vi "make_axes_caption.vi"(7 "Caption Properties":T2={"Show Captions"={"Show X Caption"=FALSE, "Show Z Caption"=TRUE, "Show Y Caption"=TRUE, "Show Opposite X Caption"=FALSE, "Show Opposite Y Caption"=TRUE, "Show Opposite Z Caption"=TRUE}, "Captions"={"Caption X"="", "Caption Y"="", "Caption Z"=""}, "Caption Color"={"Color X"=0, "Color Y"=0, "Color Z"=0}, "Caption Font Size"={"Font Size X"=12, "Font Size Y"=12, "Font Size Z"=12}}, 8 "Length":dbl, 9 "View Direction":T1(ring), 10 "Label Width":T3, 11 "Scene Object In":refnum<vi>) -> (3 "Scene Object Out":refnum<vi>)   [LabVIEW 2020, in "3DPC_SurfacePlot.xctl"]
uses:
  <vilib>/Native 3D Graph/xcontrol/3DPC_SurfacePlot.xctl
  <vilib>/Native 3D Graph/typedefs/prop_axes_captions.ctl
  <vilib>/Utility/miscctls.llb/LV3DPointTypeDef.ctl
  <vilib>/picture/3D Picture Control/Object/Create Object (name).vi
  <vilib>/picture/3D Picture Control/NI_3D Picture Control.lvlib
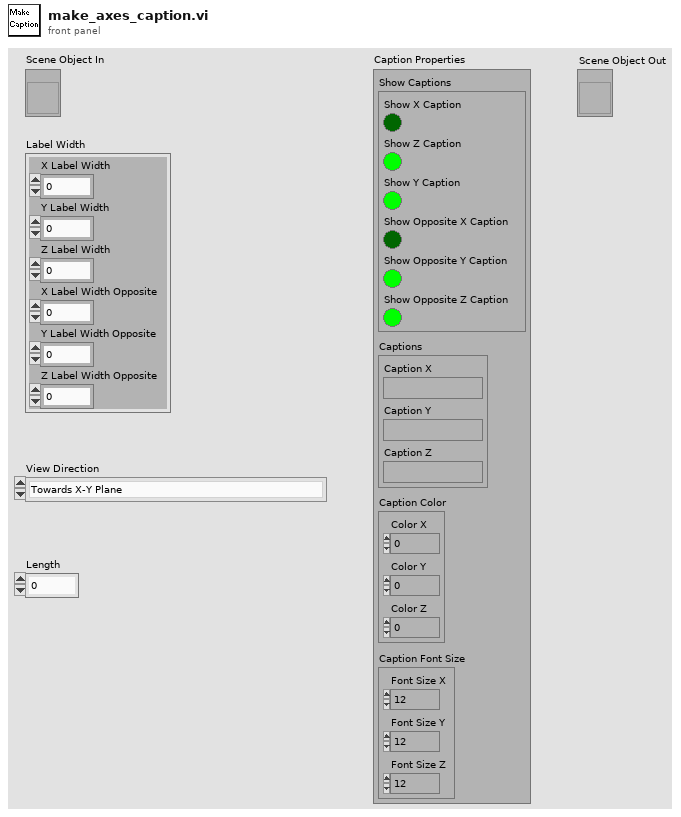
[diagram p1: front panel]
types:
  T1 = enum32{"Towards X-Y Plane", "Towards Y-Z Plane", "Towards X-Z Plane", "User Define"}
  T2 = typedef "3DPC_SurfacePlot.xctl/prop_axes_captions.ctl" = cluster{"Show Captions":cluster{"Show X Caption":bool, "Show Z Caption":bool, "Show Y Caption":bool, "Show Opposite X Caption":bool, "Show Opposite Y Caption":bool, "Show Opposite Z Caption":bool}, "Captions":cluster{"Caption X":string, "Caption Y":string, "Caption Z":string}, "Caption Color":cluster{"Color X":u32, "Color Y":u32, "Color Z":u32}, "Caption Font Size":cluster{"Font Size X":i16, "Font Size Y":i16, "Font Size Z":i16}}
  T3 = cluster{"X Label Width":dbl, "Y Label Width":dbl, "Z Label Width":dbl, "X Label Width Opposite":dbl, "Y Label Width Opposite":dbl, "Z Label Width Opposite":dbl}
  T4 = cluster{"Show X Caption":bool, "Show Z Caption":bool, "Show Y Caption":bool, "Show Opposite X Caption":bool, "Show Opposite Y Caption":bool, "Show Opposite Z Caption":bool}
  T5 = cluster{"Caption X":string, "Caption Y":string, "Caption Z":string}
  T6 = cluster{"Font Size X":i16, "Font Size Y":i16, "Font Size Z":i16}
  T7 = cluster{"Font Size X":dbl, "Font Size Y":dbl, "Font Size Z":dbl}
  T8 = typedef "LV3DPointTypeDef.ctl" = cluster{"X":sgl, "Y":sgl, "Z":sgl}
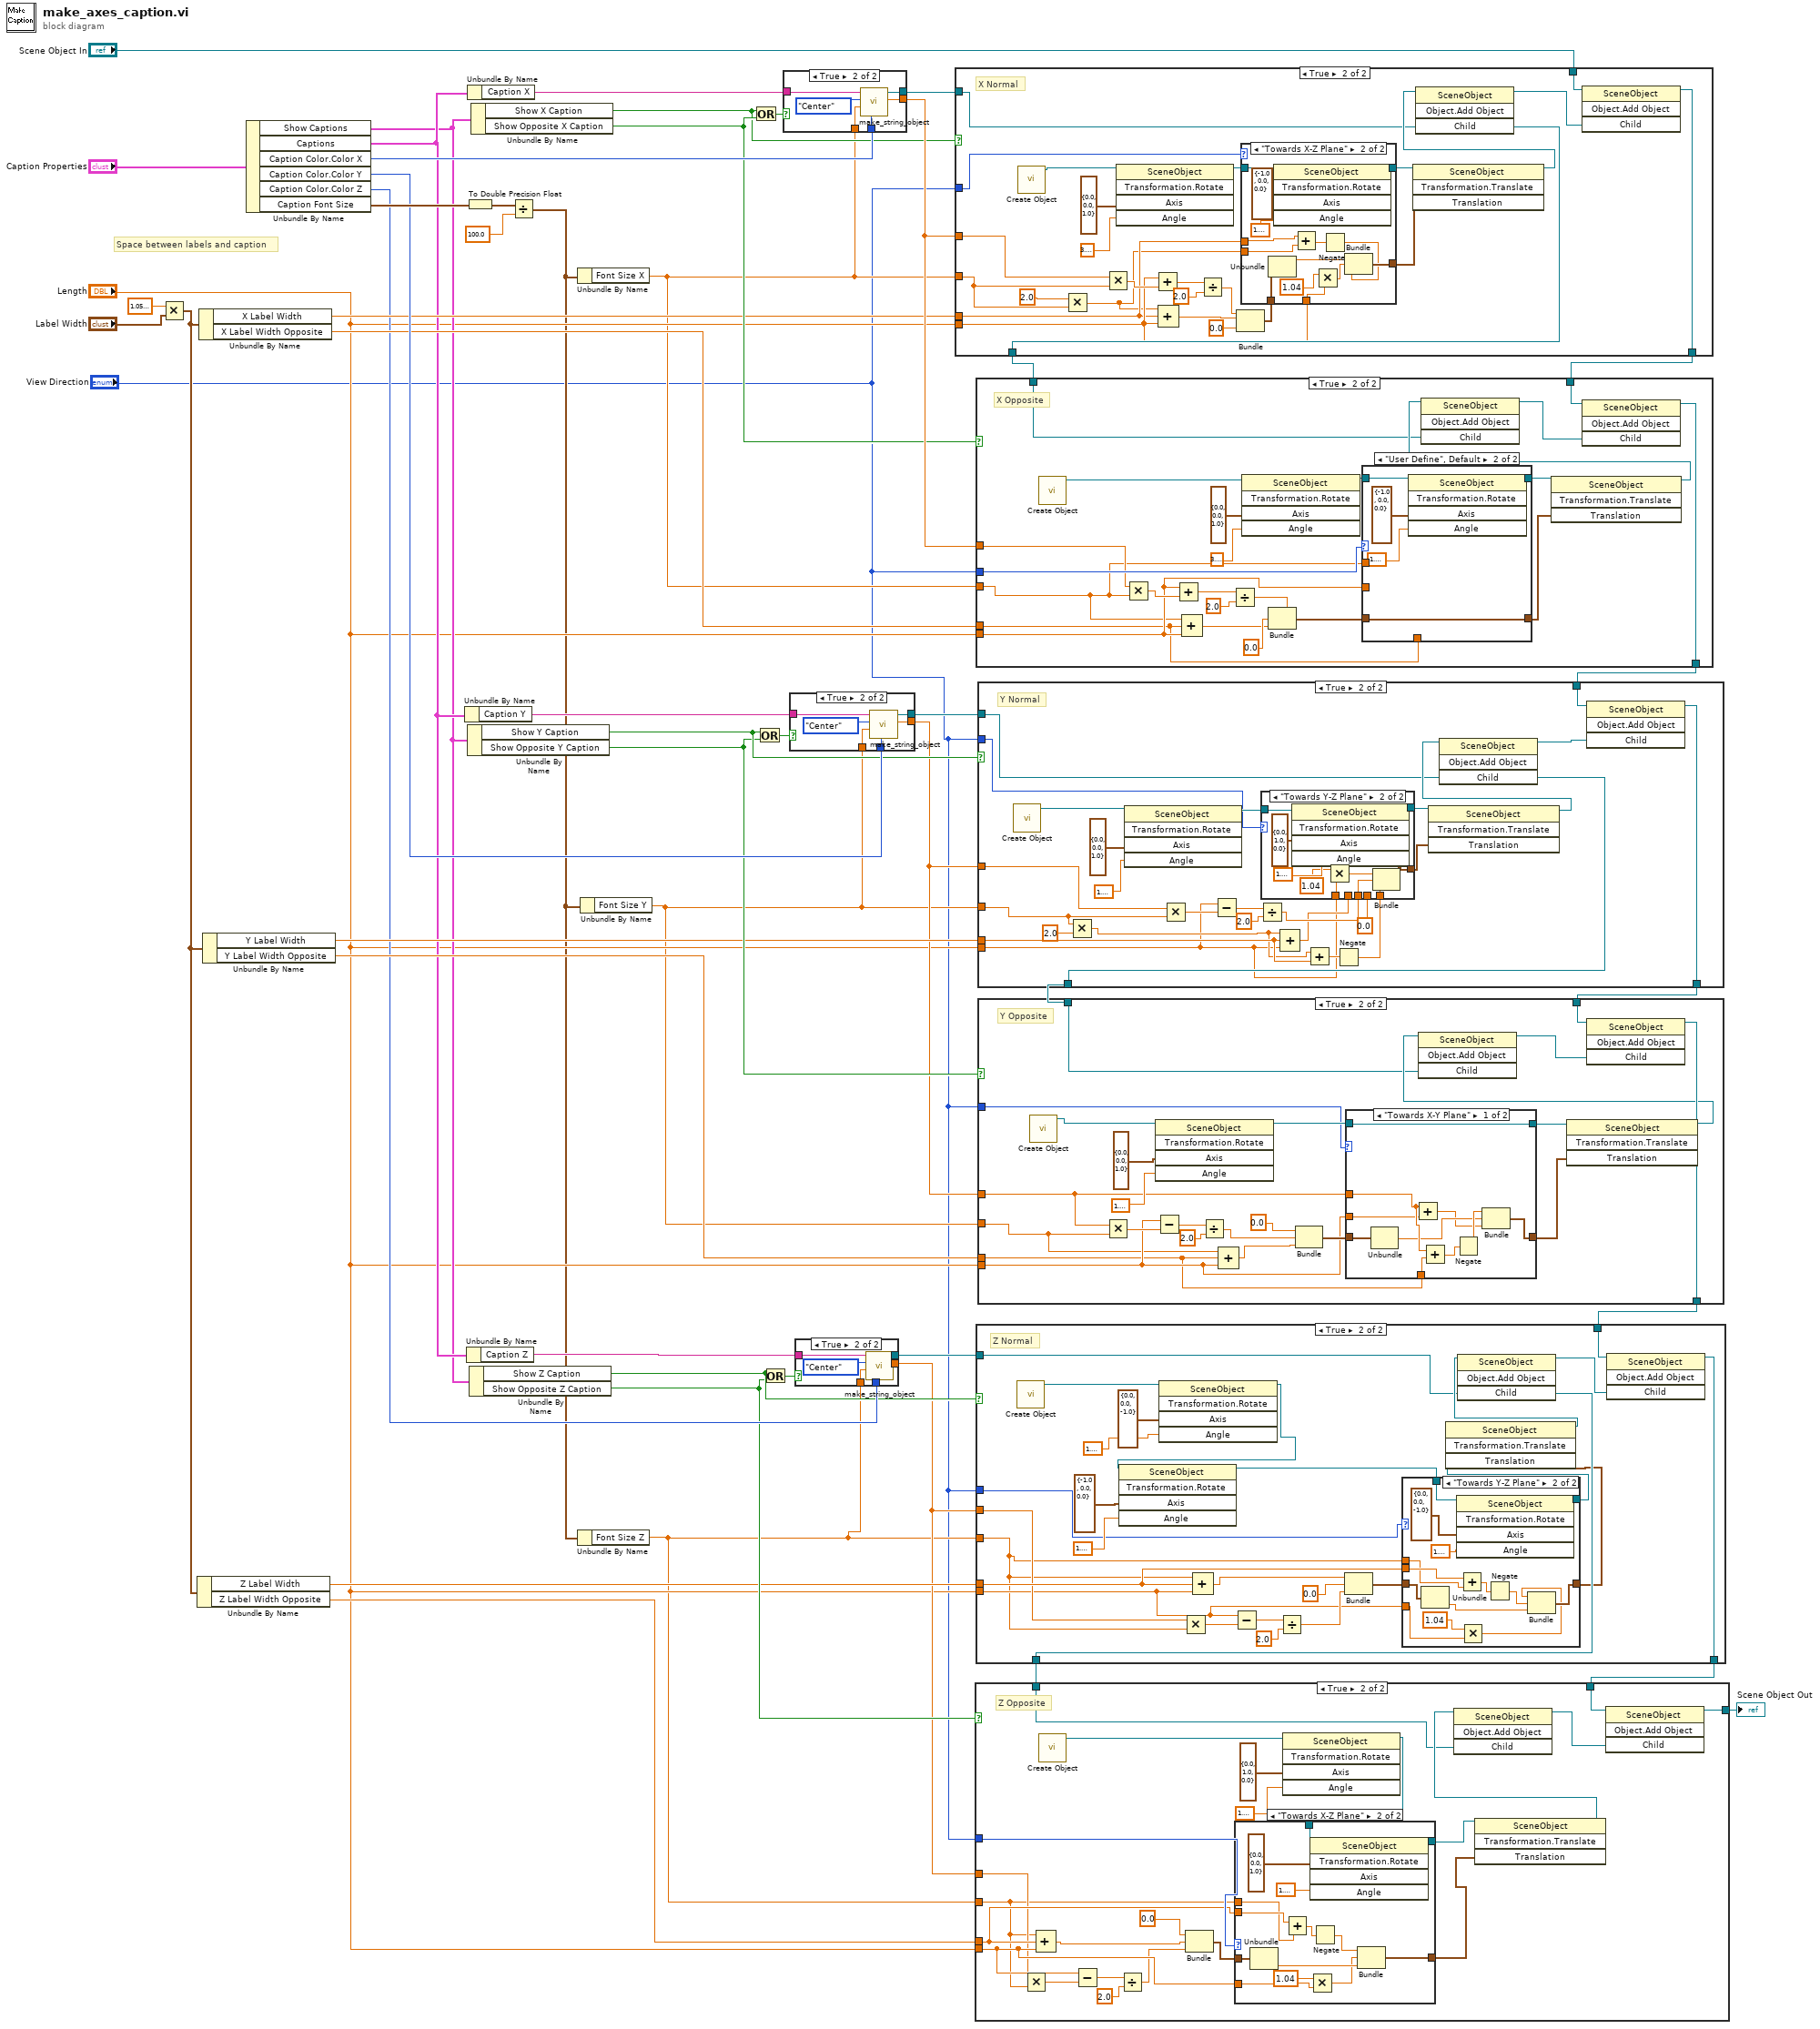
[diagram p0: block diagram]
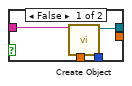
[diagram p2: hidden frame]
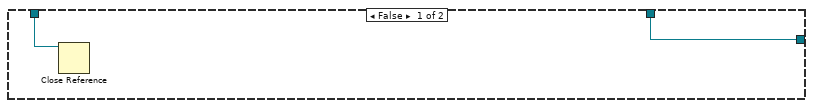
[diagram p3: hidden frame]
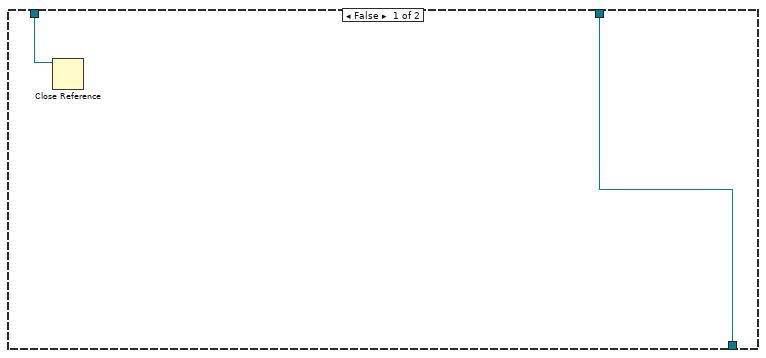
[diagram p5: hidden frame]
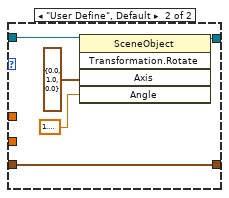
[diagram p6: hidden frame]
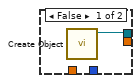
[diagram p7: hidden frame]
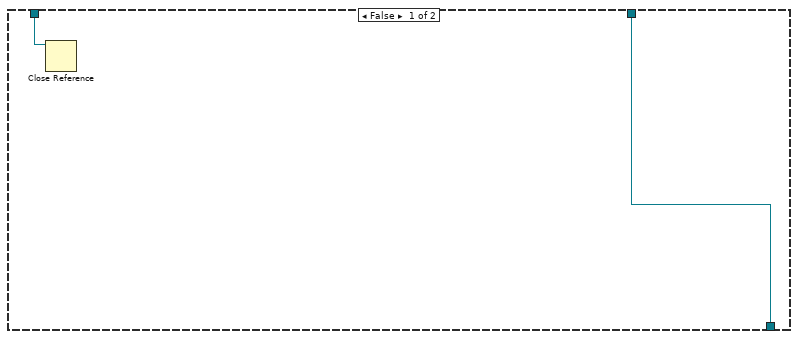
[diagram p8: hidden frame]
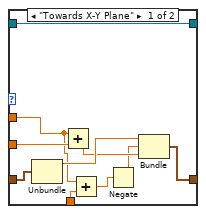
[diagram p9: hidden frame]
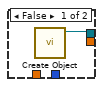
[diagram p10: hidden frame]
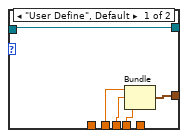
[diagram p14: hidden frame]
diagram:
  # "Space between labels and caption"
  n1 = Multiply(x=sgl 1.06, y="Label Width") -> (x*y=w2:T3)
  n2 = Unbundle By Name(w2) -> ("Z Label Width"=w15:dbl, "Z Label Width Opposite"=w14:dbl)
  n3 = Unbundle By Name(w2) -> ("X Label Width"=w35:dbl, "X Label Width Opposite"=w34:dbl)
  n4 = Unbundle By Name(w2) -> ("Y Label Width"=w28:dbl, "Y Label Width Opposite"=w27:dbl)
  n5 = Unbundle By Name("Caption Properties") -> ("Show Captions"=w20:T4, "Captions"=w21:T5, "Caption Color.Color X"=w48:u32, "Caption Color.Color Y"=w40:u32, "Caption Color.Color Z"=w19:u32, "Caption Font Size"=w49:T6)
  n6 = Unbundle By Name(w21) -> ("Caption Y"=w36:string)
  n7 = To Double Precision Float(number=w49) -> (double precision float=w8:T7)
  n8 = Unbundle By Name(w21) -> ("Caption Z"=w22:string)
  n9 = Unbundle By Name(w21) -> ("Caption X"=w37:string)
  n10 = Unbundle By Name(w20) -> ("Show Y Caption"=w33:bool, "Show Opposite Y Caption"=w29:bool)
  n11 = Unbundle By Name(w20) -> ("Show Z Caption"=w17:bool, "Show Opposite Z Caption"=w16:bool)
  n12 = Unbundle By Name(w20) -> ("Show X Caption"=w38:bool, "Show Opposite X Caption"=w41:bool)
  n13 = Divide(x=w8, y=100.0) -> (x/y=w4:T7)
  n14 = Unbundle By Name(w4) -> ("Font Size X"=w7:dbl)
  n15 = Unbundle By Name(w4) -> ("Font Size Z"=w5:dbl)
  n16 = Unbundle By Name(w4) -> ("Font Size Y"=w6:dbl)
  n17 = Or(x=w38, y=w41) -> (x .or. y?=w47:bool)
  n18 = Or(x=w33, y=w29) -> (x .or. y?=w39:bool)
  n19 = Or(x=w17, y=w16) -> (x .or. y?=w18:bool)
  n20 = case shown="True" w47 {
    tunnel: w37 -> [_ w59]
    tunnel: w48 -> [_ w58]
    tunnel: [w53 w57] -> w46
    tunnel: [_ w56] -> w42
    tunnel: w7 -> [_ w54]
    frame False {
      n21 = call-poly <vilib>:"Create Object.vi"() -> ("Scene:New Object"=w53:refnum<vi>)  [unwired: 10 in, 1 out]
    }
    frame True {
      n22 = call <vilib>:"make_string_object.vi"("Color"=w58, "Font Size"=w54, "Alignment:Horizontal"=enum8{"Left", "Right", "Center"}."Center", "String"=w59) -> ("Width"=w56:dbl, "String Object Out"=w57:refnum<vi>)  [unwired: 6 out]
    }
  }
  n23 = case shown="True" w39 {
    tunnel: w36 -> [_ w66]
    tunnel: [w60 w65] -> w30
    tunnel: [_ w64] -> w26
    tunnel: w40 -> [_ w63]
    tunnel: w6 -> [_ w61]
    frame False {
      n24 = call-poly <vilib>:"Create Object.vi"() -> ("Scene:New Object"=w60:refnum<vi>)  [unwired: 10 in, 1 out]
    }
    frame True {
      n25 = call <vilib>:"make_string_object.vi"("Color"=w63, "Font Size"=w61, "Alignment:Horizontal"=enum8{"Left", "Right", "Center"}."Center", "String"=w66) -> ("Width"=w64:dbl, "String Object Out"=w65:refnum<vi>)  [unwired: 6 out]
    }
  }
  n26 = case shown="True" w18 {
    tunnel: w22 -> [w68 w74]
    tunnel: [w67 w73] -> w12
    tunnel: [_ w72] -> w13
    tunnel: w19 -> [_ w71]
    tunnel: w5 -> [_ w69]
    frame False {
      n27 = call-poly <vilib>:"Create Object.vi"("Name"=w68) -> ("Scene:New Object"=w67:refnum<vi>)  [unwired: 9 in, 1 out]
    }
    frame True {
      n28 = call <vilib>:"make_string_object.vi"("Color"=w71, "Font Size"=w69, "Alignment:Horizontal"=enum8{"Left", "Right", "Center"}."Center", "String"=w74) -> ("Width"=w72:dbl, "String Object Out"=w73:refnum<vi>)  [unwired: 6 out]
    }
  }
  n29 = case shown="True" w38 {
    tunnel: "Scene Object In" -> [w76 w100]
    tunnel: w7 -> [_ w78]
    tunnel: w35 -> [_ w80]
    tunnel: "Length" -> [_ w83]
    tunnel: [w76 w99] -> w45
    tunnel: w46 -> [w75 w92]
    tunnel: w42 -> [_ w81]
    tunnel: [w75 w94] -> w43
    tunnel: "View Direction" -> [_ w87]
    frame False {
    }
    frame True {
      # "X Normal"
      n30 = call-poly <vilib>:"Create Object.vi"() -> ("Scene:New Object"=w91:refnum<vi>)  [unwired: 10 in, 1 out]
      n31 = Multiply(x=2.0, y=w78) -> (x*y=w77:dbl)
      n32 = Multiply(x=w81, y=w78) -> (x*y=w98:dbl)
      n33 = invoke class="SceneObject" method="Transformation.Rotate"(reference=w91, "Axis"=cluster{"X":sgl, "Y":sgl, "Z":sgl} {"X"=0.0, "Y"=0.0, "Z"=1.0}, "Angle"=3.141592653589793) -> (reference out=w89:refnum<vi>)  [unwired: 2 in, 4 out]
      n34 = Add(x=w83, y=w98) -> (x+y=w97:dbl)
      n35 = Compound Arithmetic op=ADD(w77, w80, w83) -> (w86:dbl)
      n36 = Divide(x=w97, y=2.0) -> (x/y=w90:dbl)
      n37 = Bundle(w90, w86, "y"=0.0) -> (w85:cluster{dbl, dbl, "y":dbl})  [unwired: 1 out]
      n38 = case shown="\"Towards X-Z Plane\"" w87 {
        tunnel: w89 -> [w104 w118]
        tunnel: [w104 w117] -> w88
        tunnel: w85 -> [w103 w114]
        tunnel: [w103 w112] -> w84
        tunnel: w83 -> [_ w107]
        tunnel: w77 -> [_ w110]
        tunnel: w80 -> [_ w111]
        frame "User Define", Default {
        }
        frame "Towards X-Z Plane" {
          n39 = Unbundle(w114) -> (w113:dbl)  [unwired: 2 out]
          n40 = invoke class="SceneObject" method="Transformation.Rotate"(reference=w118, "Axis"=T8 {"X"=-1.0, "Y"=0.0, "Z"=0.0}, "Angle"=1.5707963267948966) -> (reference out=w117:refnum<vi>)  [unwired: 2 in, 4 out]
          n41 = Add(x=w111, y=w110) -> (x+y=w109:dbl)
          n42 = Multiply(x=1.04 ("y"), y=w107) -> (x*y=w105:dbl)
          n43 = Negate(x=w109) -> (-x=w108:dbl)
          n44 = Bundle(w113, w105, w108) -> (w112:cluster{dbl, dbl, dbl})  [unwired: 1 out]
        }
      }
      n45 = invoke class="SceneObject" method="Transformation.Translate"(reference=w88, "Translation"=w84) -> (reference out=w93:refnum<vi>)  [unwired: 2 in, 3 out]
      n46 = invoke class="SceneObject" method="Object.Add Object"(reference=w93, "Child"=w92) -> (reference out=w95:refnum<vi>, "Child"=w94:refnum<vi>)  [unwired: 2 in, 2 out]
      n47 = invoke class="SceneObject" method="Object.Add Object"(reference=w100, "Child"=w95) -> (reference out=w99:refnum<vi>)  [unwired: 2 in, 3 out]
    }
  }
  n48 = case shown="True" w41 {
    tunnel: w45 -> [w120 w141]
    tunnel: w7 -> [_ w121]
    tunnel: w34 -> [_ w122]
    tunnel: [w120 w140] -> w44
    tunnel: w42 -> [_ w124]
    tunnel: w43 -> [w119 w133]
    tunnel: "Length" -> [_ w123]
    tunnel: "View Direction" -> [_ w127]
    frame False {
      n49 = Close Reference(reference=w119) -> ()  [unwired: 1 in, 1 out]
    }
    frame True {
      # "X Opposite"
      n50 = call-poly <vilib>:"Create Object.vi"() -> ("Scene:New Object"=w128:refnum<vi>)  [unwired: 10 in, 1 out]
      n51 = Multiply(x=w124, y=w121) -> (x*y=w139:dbl)
      n52 = Add(x=w123, y=w139) -> (x+y=w138:dbl)
      n53 = Compound Arithmetic op=ADD(w121, w122, w123) -> (w129:dbl)
      n54 = Divide(x=w138, y=2.0) -> (x/y=w136:dbl)
      n55 = invoke class="SceneObject" method="Transformation.Rotate"(reference=w128, "Axis"=cluster{"X":sgl, "Y":sgl, "Z":sgl} {"X"=0.0, "Y"=0.0, "Z"=1.0}, "Angle"=3.141592653589793) -> (reference out=w132:refnum<vi>)  [unwired: 2 in, 4 out]
      n56 = Bundle(w136, "x+y"=0.0, w129) -> (w126:cluster{dbl, "x+y":dbl, dbl})  [unwired: 1 out]
      n57 = case shown="\"User Define\", Default" w127 {
        tunnel: w132 -> [w153 w158]
        tunnel: [w153 w157] -> w131
        tunnel: w126 -> [w152 w154]
        tunnel: [w151 w154] -> w125
        tunnel: w121 -> [w146 _]
        tunnel: w123 -> [w149 _]
        tunnel: w122 -> [w147 _]
        frame "Towards X-Y Plane" {
          n58 = Unbundle(w152) -> (w150:dbl)  [unwired: 2 out]
          n59 = Add(x=w146, y=w149) -> (x+y=w148:dbl)
          n60 = Add(x=w146, y=w147) -> (x+y=w145:dbl)
          n61 = Negate(x=w145) -> (-x=w144:dbl)
          n62 = Bundle(w150, w144, w148) -> (w151:cluster{dbl, dbl, dbl})  [unwired: 1 out]
        }
        frame "User Define", Default {
          n63 = invoke class="SceneObject" method="Transformation.Rotate"(reference=w158, "Axis"=cluster{"X":sgl, "Y":sgl, "Z":sgl} {"X"=-1.0, "Y"=0.0, "Z"=0.0}, "Angle"=1.5707963267948966) -> (reference out=w157:refnum<vi>)  [unwired: 2 in, 4 out]
        }
      }
      n64 = invoke class="SceneObject" method="Transformation.Translate"(reference=w131, "Translation"=w125) -> (reference out=w134:refnum<vi>)  [unwired: 2 in, 3 out]
      n65 = invoke class="SceneObject" method="Object.Add Object"(reference=w134, "Child"=w133) -> (reference out=w135:refnum<vi>)  [unwired: 2 in, 3 out]
      n66 = invoke class="SceneObject" method="Object.Add Object"(reference=w141, "Child"=w135) -> (reference out=w140:refnum<vi>)  [unwired: 2 in, 3 out]
    }
  }
  n67 = case shown="True" w33 {
    tunnel: w6 -> [_ w163]
    tunnel: w28 -> [_ w168]
    tunnel: "Length" -> [_ w161]
    tunnel: w44 -> [w160 w186]
    tunnel: [w160 w185] -> w32
    tunnel: w26 -> [_ w166]
    tunnel: w30 -> [w159 w178]
    tunnel: [w159 w177] -> w25
    tunnel: "View Direction" -> [_ w173]
    frame False {
    }
    frame True {
      # "Y Normal"
      n68 = call-poly <vilib>:"Create Object.vi"() -> ("Scene:New Object"=w176:refnum<vi>)  [unwired: 10 in, 1 out]
      n69 = Multiply(x=w163, y=2.0) -> (x*y=w164:dbl)
      n70 = invoke class="SceneObject" method="Transformation.Rotate"(reference=w176, "Axis"=cluster{"X":sgl, "Y":sgl, "Z":sgl} {"X"=0.0, "Y"=0.0, "Z"=1.0}, "Angle"=1.5707963267948966) -> (reference out=w175:refnum<vi>)  [unwired: 2 in, 4 out]
      n71 = Multiply(x=w166, y=w163) -> (x*y=w184:dbl)
      n72 = Subtract(x=w161, y=w184) -> (x-y=w183:dbl)
      n73 = Divide(x=w183, y=2.0) -> (x/y=w172:dbl)
      n74 = Compound Arithmetic op=ADD(w164, w168, w161) -> (w169:dbl)
      n75 = Add(x=w164, y=w168) -> (x+y=w167:dbl)
      n76 = Negate(x=w167) -> (-x=w170:dbl)
      n77 = case shown="\"Towards Y-Z Plane\"" w173 {
        tunnel: w175 -> [w192 w202]
        tunnel: [w192 w201] -> w174
        tunnel: w169 -> [w191 _]
        tunnel: w172 -> [w190 w197]
        tunnel: 0.0 ("y") -> [w189 _]
        tunnel: [w188 w198] -> w171
        tunnel: w170 -> [_ w196]
        tunnel: w161 -> [_ w194]
        frame "User Define", Default {
          n78 = Bundle(w191, w190, "y"=w189) -> (w188:cluster{dbl, dbl, "y":dbl})  [unwired: 1 out]
        }
        frame "Towards Y-Z Plane" {
          n79 = invoke class="SceneObject" method="Transformation.Rotate"(reference=w202, "Axis"=T8 {"X"=0.0, "Y"=1.0, "Z"=0.0}, "Angle"=1.5707963267948966) -> (reference out=w201:refnum<vi>)  [unwired: 2 in, 4 out]
          n80 = Multiply(x=1.04 ("y"), y=w194) -> (x*y=w193:dbl)
          n81 = Bundle(w193, w197, w196) -> (w198:cluster{dbl, dbl, dbl})  [unwired: 1 out]
        }
      }
      n82 = invoke class="SceneObject" method="Transformation.Translate"(reference=w174, "Translation"=w171) -> (reference out=w180:refnum<vi>)  [unwired: 2 in, 3 out]
      n83 = invoke class="SceneObject" method="Object.Add Object"(reference=w180, "Child"=w178) -> (reference out=w179:refnum<vi>, "Child"=w177:refnum<vi>)  [unwired: 2 in, 2 out]
      n84 = invoke class="SceneObject" method="Object.Add Object"(reference=w186, "Child"=w179) -> (reference out=w185:refnum<vi>)  [unwired: 2 in, 3 out]
    }
  }
  n85 = case shown="True" w29 {
    tunnel: w6 -> [_ w205]
    tunnel: w27 -> [_ w206]
    tunnel: "Length" -> [_ w207]
    tunnel: w32 -> [w204 w226]
    tunnel: [w204 w225] -> w31
    tunnel: w26 -> [_ w208]
    tunnel: w25 -> [w203 w217]
    tunnel: "View Direction" -> [_ w211]
    frame False {
      n86 = Close Reference(reference=w203) -> ()  [unwired: 1 in, 1 out]
    }
    frame True {
      # "Y Opposite"
      n87 = call-poly <vilib>:"Create Object.vi"() -> ("Scene:New Object"=w212:refnum<vi>)  [unwired: 10 in, 1 out]
      n88 = Multiply(x=w208, y=w205) -> (x*y=w224:dbl)
      n89 = invoke class="SceneObject" method="Transformation.Rotate"(reference=w212, "Axis"=cluster{"X":sgl, "Y":sgl, "Z":sgl} {"X"=0.0, "Y"=0.0, "Z"=1.0}, "Angle"=1.5707963267948966) -> (reference out=w214:refnum<vi>)  [unwired: 2 in, 4 out]
      n90 = Subtract(x=w207, y=w224) -> (x-y=w223:dbl)
      n91 = Divide(x=w223, y=2.0) -> (x/y=w221:dbl)
      n92 = Compound Arithmetic op=ADD(w205, w206, w207) -> (w216:dbl)
      n93 = Bundle("x+y"=0.0, w221, w216) -> (w210:cluster{"x+y":dbl, dbl, dbl})  [unwired: 1 out]
      n94 = case shown="\"Towards X-Y Plane\"" w211 {
        tunnel: w214 -> [w237 w242]
        tunnel: [w237 w241] -> w213
        tunnel: w210 -> [w234 w238]
        tunnel: [w235 w238] -> w209
        tunnel: w208 -> [w233 _]
        tunnel: w207 -> [w232 _]
        tunnel: w206 -> [w231 _]
        frame "Towards X-Y Plane" {
          n95 = Unbundle(w234) -> (w229:dbl)  [unwired: 2 out]
          n96 = Add(x=w233, y=w232) -> (x+y=w228:dbl)
          n97 = Add(x=w233, y=w231) -> (x+y=w236:dbl)
          n98 = Negate(x=w236) -> (-x=w230:dbl)
          n99 = Bundle(w230, w229, w228) -> (w235:cluster{dbl, dbl, dbl})  [unwired: 1 out]
        }
        frame "User Define", Default {
          n100 = invoke class="SceneObject" method="Transformation.Rotate"(reference=w242, "Axis"=cluster{"X":sgl, "Y":sgl, "Z":sgl} {"X"=0.0, "Y"=1.0, "Z"=0.0}, "Angle"=1.5707963267948966) -> (reference out=w241:refnum<vi>)  [unwired: 2 in, 4 out]
        }
      }
      n101 = invoke class="SceneObject" method="Transformation.Translate"(reference=w213, "Translation"=w209) -> (reference out=w219:refnum<vi>)  [unwired: 2 in, 3 out]
      n102 = invoke class="SceneObject" method="Object.Add Object"(reference=w219, "Child"=w217) -> (reference out=w218:refnum<vi>)  [unwired: 2 in, 3 out]
      n103 = invoke class="SceneObject" method="Object.Add Object"(reference=w226, "Child"=w218) -> (reference out=w225:refnum<vi>)  [unwired: 2 in, 3 out]
    }
  }
  n104 = case shown="True" w17 {
    tunnel: w13 -> [_ w247]
    tunnel: w15 -> [_ w248]
    tunnel: "Length" -> [_ w246]
    tunnel: w31 -> [w244 w271]
    tunnel: [w244 w264] -> w23
    tunnel: w5 -> [_ w245]
    tunnel: w12 -> [w243 w262]
    tunnel: [w243 w260] -> w11
    tunnel: "View Direction" -> [_ w253]
    frame False {
    }
    frame True {
      # "Z Normal"
      n105 = call-poly <vilib>:"Create Object.vi"() -> ("Scene:New Object"=w259:refnum<vi>)  [unwired: 10 in, 1 out]
      n106 = invoke class="SceneObject" method="Transformation.Rotate"(reference=w259, "Axis"=cluster{"X":sgl, "Y":sgl, "Z":sgl} {"X"=0.0, "Y"=0.0, "Z"=-1.0}, "Angle"=1.5707963267948966) -> (reference out=w270:refnum<vi>)  [unwired: 2 in, 4 out]
      n107 = invoke class="SceneObject" method="Transformation.Rotate"(reference=w270, "Axis"=cluster{"X":sgl, "Y":sgl, "Z":sgl} {"X"=-1.0, "Y"=0.0, "Z"=0.0}, "Angle"=1.5707963267948966) -> (reference out=w252:refnum<vi>)  [unwired: 2 in, 4 out]
      n108 = Multiply(x=w247, y=w245) -> (x*y=w268:dbl)
      n109 = Compound Arithmetic op=ADD(w245, w248, w246) -> (w269:dbl)
      n110 = Subtract(x=w246, y=w268) -> (x-y=w267:dbl)
      n111 = Divide(x=w267, y=2.0) -> (x/y=w265:dbl)
      n112 = Bundle(w269, "y"=0.0, w265) -> (w250:cluster{dbl, "y":dbl, dbl})  [unwired: 1 out]
      n113 = case shown="\"Towards Y-Z Plane\"" w253 {
        tunnel: w252 -> [w273 w285]
        tunnel: [w273 w284] -> w251
        tunnel: w250 -> [w272 w283]
        tunnel: [w272 w280] -> w249
        tunnel: w248 -> [_ w281]
        tunnel: w246 -> [_ w277]
        tunnel: w245 -> [_ w274]
        frame "User Define", Default {
        }
        frame "Towards Y-Z Plane" {
          n114 = Unbundle(w283) -> (w279:dbl)  [unwired: 2 out]
          n115 = invoke class="SceneObject" method="Transformation.Rotate"(reference=w285, "Axis"=T8 {"X"=0.0, "Y"=0.0, "Z"=-1.0}, "Angle"=1.5707963267948966) -> (reference out=w284:refnum<vi>)  [unwired: 2 in, 4 out]
          n116 = Add(x=w281, y=w274) -> (x+y=w282:dbl)
          n117 = Multiply(x=1.04, y=w277) -> (x*y=w275:dbl)
          n118 = Negate(x=w282) -> (-x=w278:dbl)
          n119 = Bundle(w275, w278, w279) -> (w280:cluster{dbl, dbl, dbl})  [unwired: 1 out]
        }
      }
      n120 = invoke class="SceneObject" method="Transformation.Translate"(reference=w251, "Translation"=w249) -> (reference out=w263:refnum<vi>)  [unwired: 2 in, 3 out]
      n121 = invoke class="SceneObject" method="Object.Add Object"(reference=w263, "Child"=w262) -> (reference out=w261:refnum<vi>, "Child"=w260:refnum<vi>)  [unwired: 2 in, 2 out]
      n122 = invoke class="SceneObject" method="Object.Add Object"(reference=w271, "Child"=w261) -> (reference out=w264:refnum<vi>)  [unwired: 2 in, 3 out]
    }
  }
  n123 = case shown="True" w16 {
    tunnel: w13 -> [_ w294]
    tunnel: w14 -> [_ w298]
    tunnel: "Length" -> [_ w297]
    tunnel: w23 -> [w289 w312]
    tunnel: [w289 w311] -> w24
    tunnel: w5 -> [_ w290]
    tunnel: w11 -> [w288 w306]
    tunnel: "View Direction" -> [_ w301]
    frame False {
      n124 = Close Reference(reference=w288) -> ()  [unwired: 1 in, 1 out]
    }
    frame True {
      # "Z Opposite"
      n125 = Multiply(x=w294, y=w290) -> (x*y=w303:dbl)
      n126 = Compound Arithmetic op=ADD(w290, w298, w297) -> (w291:dbl)
      n127 = call-poly <vilib>:"Create Object.vi"() -> ("Scene:New Object"=w302:refnum<vi>)  [unwired: 10 in, 1 out]
      n128 = Subtract(x=w297, y=w303) -> (x-y=w309:dbl)
      n129 = Divide(x=w309, y=2.0) -> (x/y=w293:dbl)
      n130 = Bundle("y"=0.0, w291, w293) -> (w300:cluster{"y":dbl, dbl, dbl})  [unwired: 1 out]
      n131 = invoke class="SceneObject" method="Transformation.Rotate"(reference=w302, "Axis"=cluster{"X":sgl, "Y":sgl, "Z":sgl} {"X"=0.0, "Y"=1.0, "Z"=0.0}, "Angle"=1.5707963267948966) -> (reference out=w295:refnum<vi>)  [unwired: 2 in, 4 out]
      n132 = case shown="\"Towards X-Z Plane\"" w301 {
        tunnel: w300 -> [w314 w328]
        tunnel: [w314 w327] -> w299
        tunnel: w298 -> [_ w324]
        tunnel: w297 -> [_ w317]
        tunnel: [w313 w321] -> w296
        tunnel: w295 -> [w313 w320]
        tunnel: w290 -> [_ w318]
        frame "User Define", Default {
        }
        frame "Towards X-Z Plane" {
          n133 = Unbundle(w328) -> (w319:dbl)  [unwired: 2 out]
          n134 = Add(x=w324, y=w318) -> (x+y=w326:dbl)
          n135 = Multiply(x=1.04, y=w317) -> (x*y=w315:dbl)
          n136 = invoke class="SceneObject" method="Transformation.Rotate"(reference=w320, "Axis"=cluster{"X":sgl, "Y":sgl, "Z":sgl} {"X"=0.0, "Y"=0.0, "Z"=1.0}, "Angle"=1.5707963267948966) -> (reference out=w321:refnum<vi>)  [unwired: 2 in, 4 out]
          n137 = Negate(x=w326) -> (-x=w325:dbl)
          n138 = Bundle(w325, w315, w319) -> (w327:cluster{dbl, dbl, dbl})  [unwired: 1 out]
        }
      }
      n139 = invoke class="SceneObject" method="Transformation.Translate"(reference=w296, "Translation"=w299) -> (reference out=w307:refnum<vi>)  [unwired: 2 in, 3 out]
      n140 = invoke class="SceneObject" method="Object.Add Object"(reference=w307, "Child"=w306) -> (reference out=w305:refnum<vi>)  [unwired: 2 in, 3 out]
      n141 = invoke class="SceneObject" method="Object.Add Object"(reference=w312, "Child"=w305) -> (reference out=w311:refnum<vi>)  [unwired: 2 in, 3 out]
    }
  }
  "Scene Object Out" <- w24
